vi "FTW-Message-Construct.vi"(0 "Message":string, 11 "error in":errorcluster) -> (4 "FTW Message":refnum<class "FTW-Message.lvclass">, 15 "error out":errorcluster)   [LabVIEW 2012, in "FTW-Actor.lvlib" / "FTW-Message.lvclass"]
uses:
  FTW-Message.lvclass
panel:
  # "Inputs"
  # "Outputs"
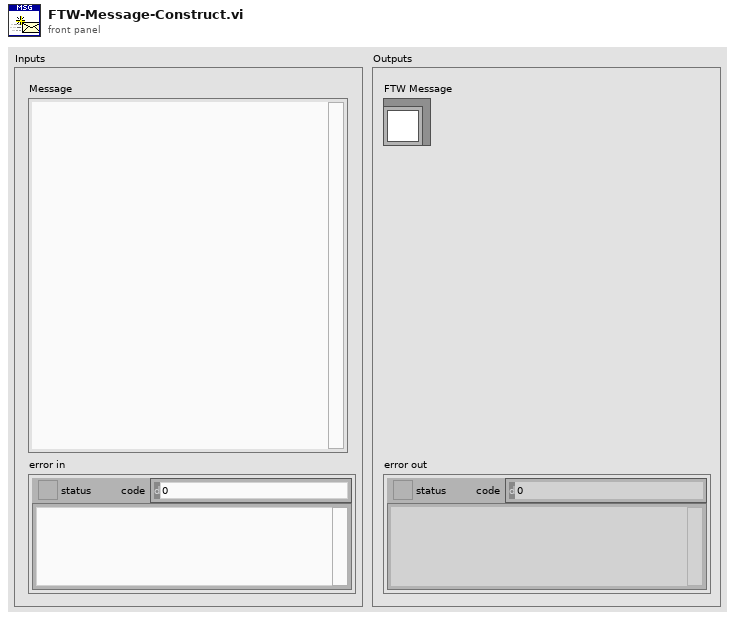
[diagram p1: front panel]
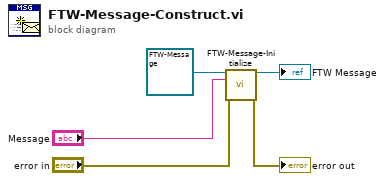
[diagram p0: block diagram]
diagram:
  n1 = call-dynamic "FTW-Message-Initialize.vi"("FTW Message"=refnum<class "FTW-Message.lvclass"> refnum, "Message"="Message", "error in"="error in") -> ("FTW Message out"=→"FTW Message":refnum<class "FTW-Message.lvclass">, "error out"=→"error out":errorcluster)  [unwired: 11 in]
